vi "signalgen.vi"(8 "error in (no error)":errorcluster, 11 "Numeric in":i32) -> (0 "error out":errorcluster, 2 "Sawtooth":dynamicdata(waveform), 3 "Numeric out":dbl)   [LabVIEW 2018, in "nn.lvlib"]
uses:
  nn.lvlib
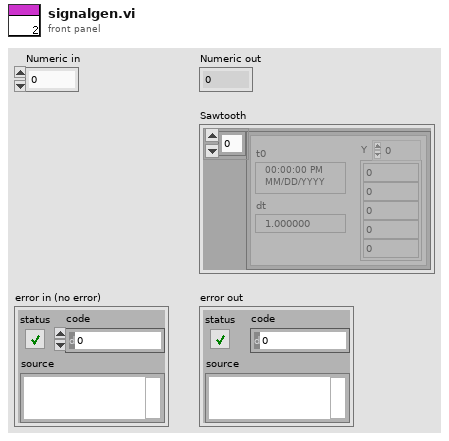
[diagram p1: front panel]
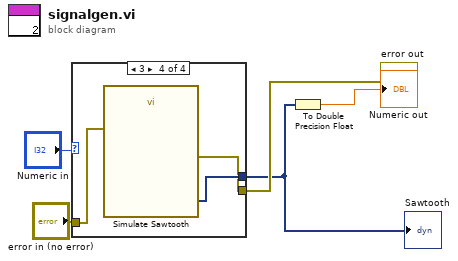
[diagram p0: block diagram]
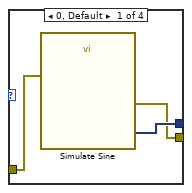
[diagram p2: hidden frame]
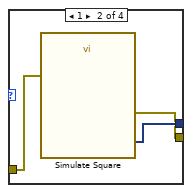
[diagram p3: hidden frame]
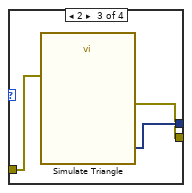
[diagram p4: hidden frame]
diagram:
  n1 = case shown="3" "Numeric in" {
    tunnel: [w8 w11 w14 w17] -> w1
    tunnel: [w7 w10 w13 w16] -> w2
    tunnel: "error in (no error)" -> [w6 w9 w12 w15]
    frame 0, Default {
      n2 = call "Simulate Sine"("error in (no error)"=w6) -> ("Sine with Uniform Noise"=w8:dynamicdata, "error out"=w7:errorcluster)  [unwired: 13 in]
    }
    frame 1 {
      n3 = call "Simulate Square"("error in (no error)"=w9) -> ("Square with Uniform Noise"=w11:dynamicdata, "error out"=w10:errorcluster)  [unwired: 13 in]
    }
    frame 2 {
      n4 = call "Simulate Triangle"("error in (no error)"=w12) -> ("Triangle with Uniform Noise"=w14:dynamicdata, "error out"=w13:errorcluster)  [unwired: 13 in]
    }
    frame 3 {
      n5 = call "Simulate Sawtooth"("error in (no error)"=w15) -> ("Sawtooth with Uniform Noise"=w17:dynamicdata, "error out"=w16:errorcluster)  [unwired: 13 in]
    }
  }
  "error out" <- w2
  "Sawtooth" <- w1
  n6 = To Double Precision Float(number=w1) -> (double precision float=→"Numeric out":dbl)
